vi "Data_GetGroup.vi"(8 "error in":errorcluster, 11 "data":variant) -> (0 "error out":errorcluster, 2 "data group":string, 3 "data out":variant)   [LabVIEW 2017, in "FileManager.lvlib"]
uses:
  <vilib>/addons/InsightCM/Devices/Shared/Common/FileManager/FileManager.lvlib
  <vilib>/addons/InsightCM/Devices/Shared/Common/FileManager/controls/DataPropertyNames.ctl
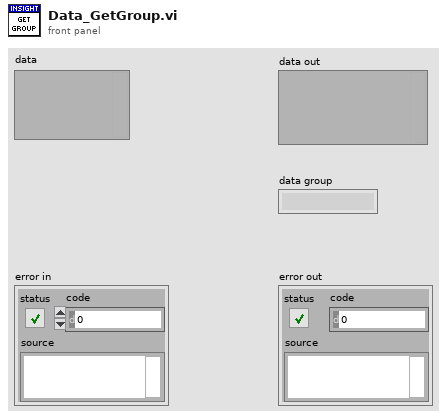
[diagram p1: front panel]
types:
  T1 = typedef "DataPropertyNames.ctl" = enum16{"Type", "EventRef", "FilePath", "DataGroup", "AcquisitionTimestamp", "StreamId", "StreamBlock", "TrendPointsOnly", "ExtraLargeFile"}
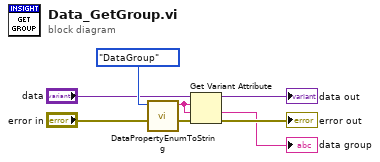
[diagram p0: block diagram]
diagram:
  n1 = call <vilib>:"DataPropertyEnumToString.vi"("property"=DataPropertyNames."DataGroup" ("Names")) -> ("string"=w2:string)  [unwired: 10 in]
  n2 = Get Variant Attribute(Variant="data", name=w2, default value (empty Variant)=w2, error in="error in") -> (duplicate Variant=→"data out":variant, value=→"data group":string, error out=→"error out":errorcluster)  [unwired: 1 out]
